vi "CleanUp Diagram.vi"(8 "error in (no error)":errorcluster, 10 "Top Level Diagram":refnum<vi>, 11 "Initial Sequence in":refnum<class "Main Sequence.lvclass">) -> (0 "error out":errorcluster, 3 "Initial Sequence out":refnum<class "Main Sequence.lvclass">)   [LabVIEW 2015, in "Main Sequence.lvclass"]
uses:
  Main Sequence.lvclass
  Structures/Structures.lvclass/Structures.ctl
  Structures/Read Structure.vi
panel:
  out "Cluster":cluster{u32, u32}
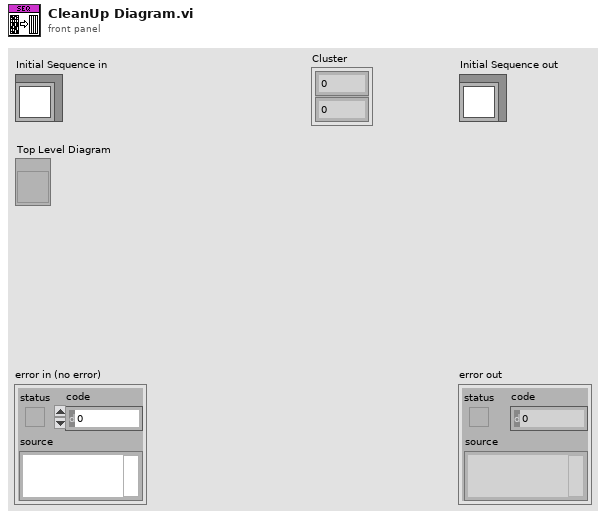
[diagram p1: front panel]
types:
  T1 = enum32{"Top Edges", "Vertical Centers", "Bottom Edges", "Left Edges", "Horizontal Centers", "Right Edges"}
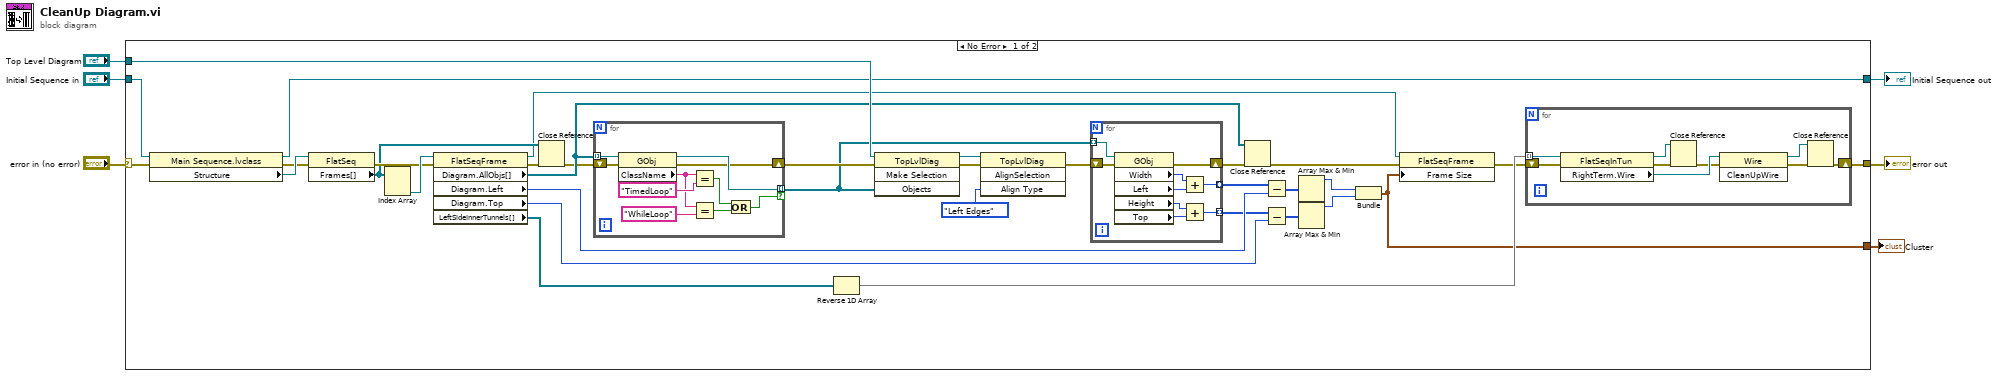
[diagram p0: block diagram]
diagram:
  n1 = case shown="No Error" "error in (no error)" {
    selector: "error in (no error)" -> [w30 w68]
    tunnel: "Initial Sequence in" -> [w31 w69]
    tunnel: "Top Level Diagram" -> [w29 _]
    tunnel: [w26 w68] -> w3
    tunnel: [w27 w69] -> w2
    tunnel: [w8 _] -> w1
    frame No Error {
      n2 = property class="Main Sequence.lvclass"(reference=w31, error in=w30) -> (reference out=w27:refnum<class "Main Sequence.lvclass">, error out=w38:errorcluster, "Structure"=w39:refnum<vi>)
      n3 = property class="FlatSeq"(reference=w39, error in=w38) -> (error out=w33:errorcluster, "Frames[]"=w21:refnum<vi>[])  [unwired: 1 out]
      n4 = Index Array(array=w21) -> (element #2=w34:refnum<vi>)  [unwired: 2 in, 1 out]
      n5 = property class="FlatSeqFrame"(reference=w34, error in=w33) -> (reference out=w7:refnum<vi>, error out=w23:errorcluster, "Diagram.AllObjs[]"=w24:refnum<vi>[], "Diagram.Left"=w18:i32, "Diagram.Top"=w17:i32, "LeftSideInnerTunnels[]"=w16:refnum<vi>[])
      n6 = Close Reference(reference=w21, error in (no error)=w23) -> (error out=w22:errorcluster)
      n7 = for {
        tunnel: w24 -> [w49] mode=indexing
        tunnel: [w44] -> w13 mode=indexing if=w40
        shift-right: [w42] -> w28
        shift-left: w22 -> [w43]
        n8 = property class="GObj"(reference=w49, error in=w43) -> (reference out=w44:refnum<vi>, error out=w42:errorcluster, "ClassName"=w41:string)
        n9 = Equal?(x=w41, y="TimedLoop") -> (x = y?=w47:bool)
        n10 = Equal?(x=w41, y="WhileLoop") -> (x = y?=w45:bool)
        n11 = Compound Arithmetic op=OR(w47, w45) -> (w40:bool)
      }
      n12 = Reverse 1D Array(array=w16) -> (reversed array=w32:refnum<vi>[])
      n13 = invoke class="TopLvlDiag" method="Make Selection"(reference=w29, error in=w28, "Objects"=w13) -> (reference out=w37:refnum<vi>, error out=w36:errorcluster)  [unwired: 1 in, 2 out]
      n14 = invoke class="TopLvlDiag" method="AlignSelection"(reference=w37, error in=w36, "Align Type"=T1."Left Edges") -> (error out=w15:errorcluster)  [unwired: 1 in, 3 out]
      n15 = for {
        tunnel: w13 -> [w58] mode=indexing
        shift-right: [w56] -> w14
        shift-left: w15 -> [w57]
        tunnel: [w53] -> w12 mode=indexing
        tunnel: [w50] -> w10 mode=indexing
        n16 = property class="GObj"(reference=w58, error in=w57) -> (error out=w56:errorcluster, "Width"=w54:u32, "Left"=w55:i32, "Height"=w52:u32, "Top"=w51:i32)  [unwired: 1 out]
        n17 = Add(x=w54, y=w55) -> (x+y=w53:u32)
        n18 = Add(x=w52, y=w51) -> (x+y=w50:u32)
      }
      n19 = Close Reference(reference=w24, error in (no error)=w14) -> (error out=w25:errorcluster)
      n20 = Subtract(x=w12, y=w18) -> (x-y=w11:u32[])
      n21 = Subtract(x=w10, y=w17) -> (x-y=w9:u32[])
      n22 = Array Max & Min(array=w11) -> (max value=w20:u32)  [unwired: 3 out]
      n23 = Array Max & Min(array=w9) -> (max value=w19:u32)  [unwired: 3 out]
      n24 = Bundle(w20, w19) -> (w8:cluster{u32, u32})  [unwired: 1 in]
      n25 = property class="FlatSeqFrame"(reference=w7, "Frame Size"=w8) -> ()  [unwired: 1 in, 2 out]
      n26 = for {
        tunnel: w32 -> [w67] mode=indexing
        shift-right: [w59] -> w26
        shift-left: w25 -> [w66]
        n27 = property class="FlatSeqInTun"(reference=w67, error in=w66) -> (reference out=w63:refnum<vi>, error out=w64:errorcluster, "RightTerm.Wire"=w65:refnum<vi>)
        n28 = Close Reference(reference=w63, error in (no error)=w64) -> (error out=w62:errorcluster)
        n29 = invoke class="Wire" method="CleanUpWire"(reference=w65, error in=w62) -> (reference out=w60:refnum<vi>, error out=w61:errorcluster)  [unwired: 1 in, 1 out]
        n30 = Close Reference(reference=w60, error in (no error)=w61) -> (error out=w59:errorcluster)
      }
    }
    frame Error {
    }
  }
  "error out" <- w3
  "Initial Sequence out" <- w2
  "Cluster" <- w1
